vi "Create.vi"(8 "error in (no error)":errorcluster, 11 "Config XML":string) -> (0 "error out":errorcluster, 3 "reference out":refnum<class "ViPER.lvclass">)   [LabVIEW 2022 SP3, in "ViPER.lvlib" / "ViPER.lvclass"]
doc: "### BSD License (http://www.opensource.org/licenses/bsd-license.php) Begin ###\n\nCopyright (c) 2018 Kurt Friday www.medulla.net\n\nAll rights reserved.\n\nRedistribution and use in source and binary forms, with or without\nmodification, are permitted provided that the following conditions are met:\n\n * Redistributions of source code must retain the above copyright\n notice, this list of conditions and the following disclaimer.\n\n * Redistributions in binary form must reproduce the above copyright\n notice, this list of conditions and the following disclaimer in the\n documentation and/or other materials provided with the distribution.\n\n * Neither the name of the <organization> nor the\n names of its contributors may be used to endorse or promote products\n derived from this software without specific prior written permission.\n\nTHIS SOFTWARE IS PROVIDED BY THE COPYRIGHT HOLDERS AND CONTRIBUTORS \"AS IS\" AND\nANY EXPRESS OR IMPLIED WARRANTIES, INCLUDING, BUT NOT LIMITED TO, THE IMPLIED\nWARRANTIES OF MERCHANTABILITY AND FITNESS FOR A PARTICULAR PURPOSE ARE\nDISCLAIMED. IN NO EVENT SHALL <COPYRIGHT HOLDER> BE LIABLE FOR ANY\nDIRECT, INDIRECT, INCIDENTAL, SPECIAL, EXEMPLARY, OR CONSEQUENTIAL DAMAGES\n(INCLUDING, BUT NOT LIMITED TO, PROCUREMENT OF SUBSTITUTE GOODS OR SERVICES;\nLOSS OF USE, DATA, OR PROFITS; OR BUSINESS INTERRUPTION) HOWEVER CAUSED AND\nON ANY THEORY OF LIABILITY, WHETHER IN CONTRACT, STRICT LIABILITY, OR TORT\n(INCLUDING NEGLIGENCE OR OTHERWISE) ARISING IN ANY WAY OUT OF THE USE OF THIS\nSOFTWARE, EVEN IF ADVISED OF THE POSSIBILITY OF SUCH DAMAGE."
uses:
  ViPER.lvclass
  ObjectLayers.ctl
  <vilib>/Utility/LVLibp/NI_PackedLibraryUtility.lvlib
panel:
  # "### BSD License (http://www.opensource.org/licenses/bsd-license.php) Begin ###\n\nCopyright (c) 2018  Kurt Friday www.medulla.net\n\nAll rights reserved.\n\nRedistribution and use in source and binary forms, with or without\nmodification, are permitted provided that the following conditions are met:\n\n    * Redistributions of source code must retain the above copyright\n      notice, this list of conditions and the following disclaimer.\n\n    * Redistributions in binary form must reproduce the above copyright\n      notice, this list of conditions and the following disclaimer in the\n      documentation and/or other materials provided with the distribution.\n\n    * Neither the name of the <organization> nor the\n      names of its contributors may be used to endorse or promote products\n      derived from this software without specific prior written permission.\n\nTHIS SOFTWARE IS PROVIDED BY THE COPYRIGHT HOLDERS AND CONTRIBUTORS \"AS IS\" AND\nANY EXPRESS OR IMPLIED WARRANTIES, INCLUDING, BUT NOT LIMITED TO, THE IMPLIED\nWARRANTIES OF MERCHANTABILITY AND FITNESS FOR A PARTICULAR PURPOSE ARE\nDISCLAIMED. IN NO EVENT SHALL <COPYRIGHT HOLDER> BE LIABLE FOR ANY\nDIRECT, INDIRECT, INCIDENTAL, SPECIAL, EXEMPLARY, OR CONSEQUENTIAL DAMAGES\n(INCLUDING, BUT NOT LIMITED TO, PROCUREMENT OF SUBSTITUTE GOODS OR SERVICES;\nLOSS OF USE, DATA, OR PROFITS; OR BUSINESS INTERRUPTION) HOWEVER CAUSED AND\nON ANY THEORY OF LIABILITY, WHETHER IN CONTRACT, STRICT LIABILITY, OR TORT\n(INCLUDING NEGLIGENCE OR OTHERWISE) ARISING IN ANY WAY OUT OF THE USE OF THIS\nSOFTWARE, EVEN IF ADVISED OF THE POSSIBILITY OF SUCH DAMAGE."
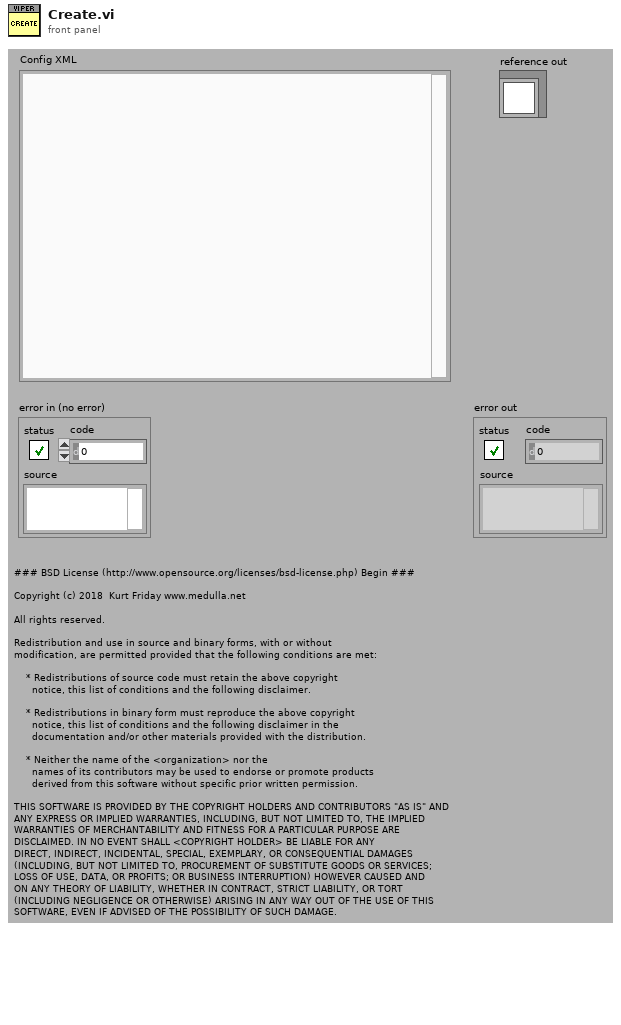
[diagram p1: front panel]
types:
  T1 = typedef "ViPER.lvlib/ViPER.lvclass/ObjectLayers.ctl" = cluster{"Ancestor":string, "Objects":refnum<class "ViPER.lvclass">[], "Object_Names":string[], "Owned":bool[]}
  T2 = typedef "ViPER.lvlib/ViPER.lvclass/ObjectDefinition.ctl" = cluster{"Name":string, "Ancestors":T3[]}
  T3 = typedef "ViPER.lvlib/ViPER.lvclass/Ancestor.ctl" = cluster{"Class":string, "Config":string, "Objects":string[]}
  T4 = typedef "ViPER.lvlib/ViPER.lvclass/Details.ctl" = cluster{"Name":string, "Class":string}
  T5 = typedef "ViPER.lvlib/ViPER.lvclass/ObjectAttributes.ctl" = cluster{"Object":T2, "Ancestors":T1[], "Config":T6, "Init_OK":bool, "Hierachy":string[], "PPL?":bool[], "SFP_Open":bool[], "Config_SFP_Open":bool[], "SoftFP_event":refnum<user-event>[], "ConfigFP_event":refnum<user-event>[], "SoftFP_Shutdown_Notifier":refnum<notifier>[], "ConfigFP_Shutdown_Notifier":refnum<notifier>[]}
  T6 = typedef "ViPER.lvlib/ViPER.lvclass/Config.ctl" = cluster{"default":string}
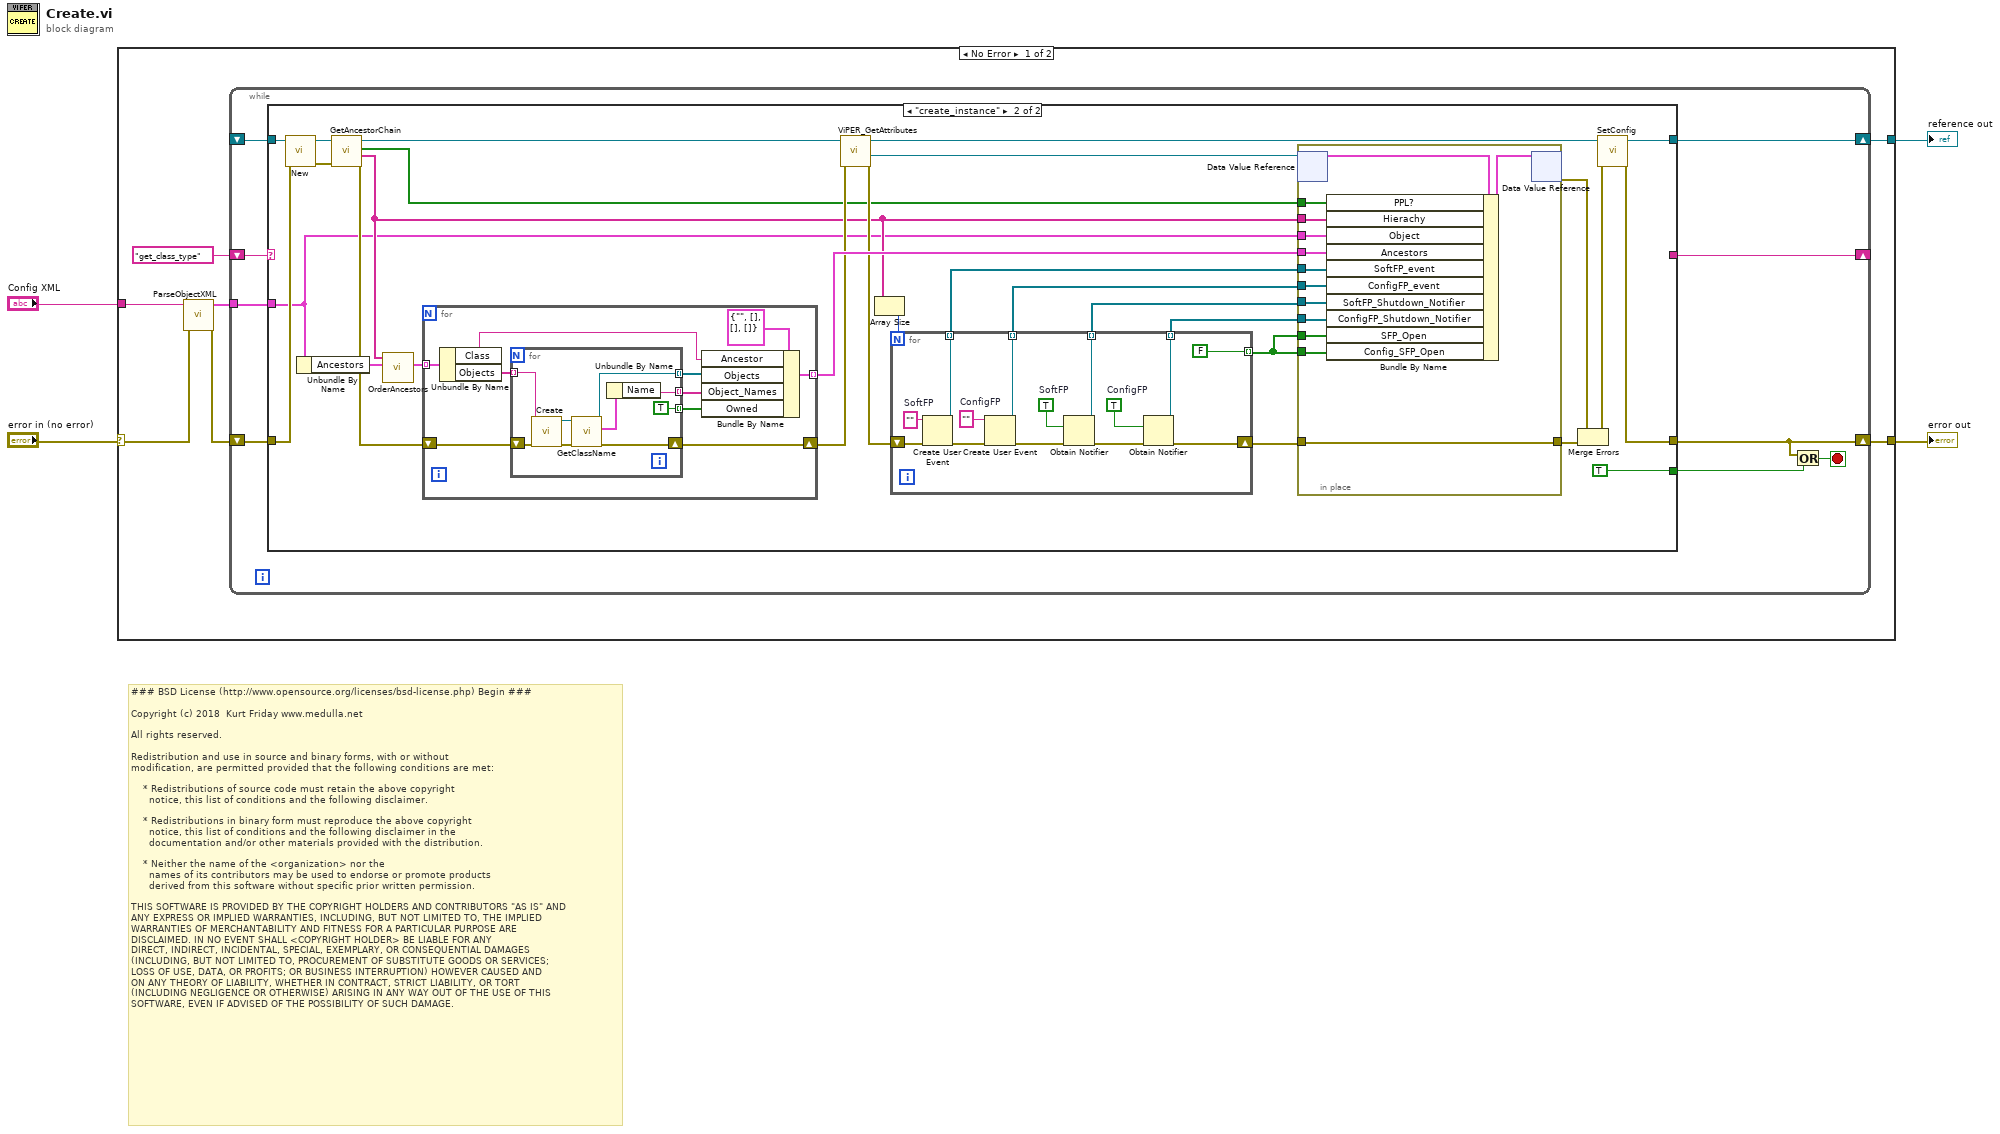
[diagram p0: block diagram]
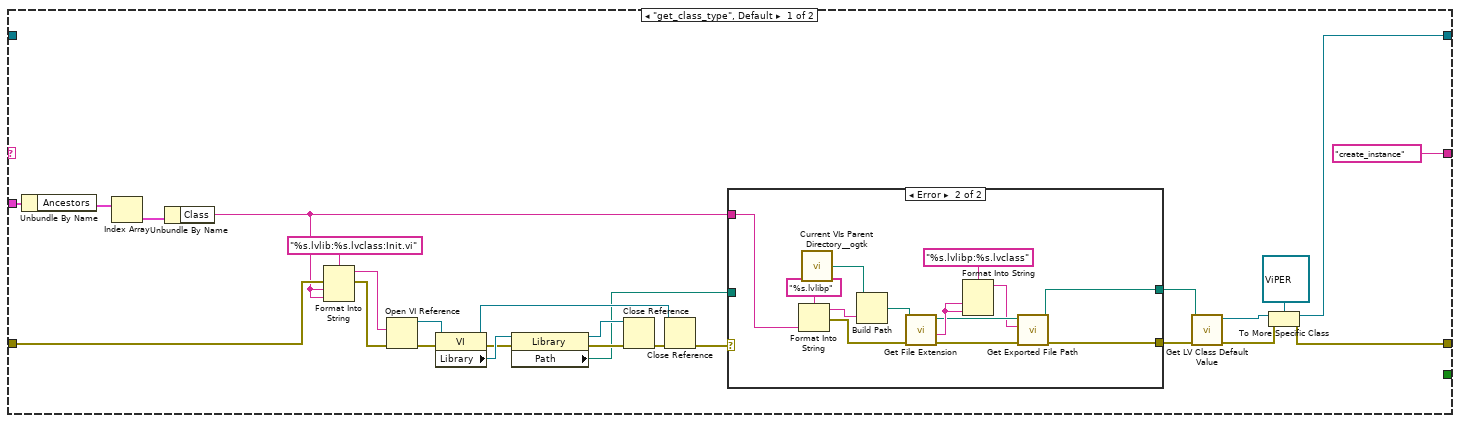
[diagram p2: hidden frame]
diagram:
  # "### BSD License (http://www.opensource.org/licenses/bsd-license.php) Begin ###\n\nCopyright (c) 2018  Kurt Friday www.medulla.net\n\nAll rights reserved.\n\nRedistribution and use in source and binary forms, with or without\nmodification, are permitted provided that the following conditions are met:\n\n    * Redistributions of source code must retain the above copyright\n      notice, this list of conditions and the following disclaimer.\n\n    * Redistributions in binary form must reproduce the above copyright\n      notice, this list of conditions and the following disclaimer in the\n      documentation and/or other materials provided with the distribution.\n\n    * Neither the name of the <organization> nor the\n      names of its contributors may be used to endorse or promote products\n      derived from this software without specific prior written permission.\n\nTHIS SOFTWARE IS PROVIDED BY THE COPYRIGHT HOLDERS AND CONTRIBUTORS \"AS IS\" AND\nANY EXPRESS OR IMPLIED WARRANTIES, INCLUDING, BUT NOT LIMITED TO, THE IMPLIED\nWARRANTIES OF MERCHANTABILITY AND FITNESS FOR A PARTICULAR PURPOSE ARE\nDISCLAIMED. IN NO EVENT SHALL <COPYRIGHT HOLDER> BE LIABLE FOR ANY\nDIRECT, INDIRECT, INCIDENTAL, SPECIAL, EXEMPLARY, OR CONSEQUENTIAL DAMAGES\n(INCLUDING, BUT NOT LIMITED TO, PROCUREMENT OF SUBSTITUTE GOODS OR SERVICES;\nLOSS OF USE, DATA, OR PROFITS; OR BUSINESS INTERRUPTION) HOWEVER CAUSED AND\nON ANY THEORY OF LIABILITY, WHETHER IN CONTRACT, STRICT LIABILITY, OR TORT\n(INCLUDING NEGLIGENCE OR OTHERWISE) ARISING IN ANY WAY OUT OF THE USE OF THIS\nSOFTWARE, EVEN IF ADVISED OF THE POSSIBILITY OF SUCH DAMAGE."
  n1 = case shown="No Error" "error in (no error)" {
    selector: "error in (no error)" -> [w8 w137]
    tunnel: "Config XML" -> [w9 _]
    tunnel: [w11 _] -> w1
    tunnel: [w10 w137] -> w2
    frame No Error {
      n2 = call "ParseObjectXML.vi"("error in (no error)"=w8, "Object XML"=w9) -> ("error out"=w7:errorcluster, "Object Cluster"=w5:T2)  [unwired: 8 in]
      n3 = while {
        shift-right: [w18] -> w10
        shift-left: w7 -> [w20]
        shift-right: [w17] -> w11
        shift-left: _ -> [w16]
        shift-right: [w15] -> _
        shift-left: "get_class_type" -> [w19]
        tunnel: w5 -> [w12]
        stop <- w13 stop-if-true
        n4 = case shown="\"create_instance\"" w19 {
          tunnel: w20 -> [w37 w84]
          tunnel: [w46 w68] -> w18
          tunnel: [w45 w70] -> w17
          tunnel: w16 -> [_ w86]
          tunnel: ["create_instance" _] -> w15
          tunnel: [_ TRUE] -> w14
          tunnel: w12 -> [w40 w64]
          frame "get_class_type", Default {
            n5 = Unbundle By Name(w40) -> ("Ancestors"=w39:T3[])
            n6 = Index Array(array=w39) -> (element=w38:T3)  [unwired: 1 in]
            n7 = Unbundle By Name(w38) -> ("Class"=w22:string)
            n8 = Format Into String(format string="%s.lvlib:%s.lvclass:Init.vi", error in=w37, w22, w22) -> (resulting string=w36:string, error out=w26:errorcluster)  [unwired: 1 in]
            n9 = Open VI Reference(vi path=w36, error in (no error)=w26) -> (vi reference=w33:refnum<vi>, error out=w28:errorcluster)  [unwired: 4 in]
            n10 = property class="VI"(reference=w33, error in=w28) -> (reference out=w35:refnum<vi>, error out=w29:errorcluster, "Library"=w30:refnum<vi>)
            n11 = property class="Library"(reference=w30, error in=w29) -> (reference out=w34:refnum<vi>, error out=w31:errorcluster, "Path"=w25:path)
            n12 = Close Reference(reference=w34, error in (no error)=w31) -> (error out=w32:errorcluster)
            n13 = Close Reference(reference=w35, error in (no error)=w32) -> (error out=w23:errorcluster)
            n14 = case shown="Error" w23 {
              selector: w23 -> [w47 _]
              tunnel: w25 -> [w48 _]
              tunnel: [w48 w50] -> w24
              tunnel: w22 -> [_ w51]
              tunnel: [w47 w49] -> w21
              frame No Error {
              }
              frame Error {
                n15 = Format Into String(format string="%s.lvlibp", w51) -> (resulting string=w60:string, error out=w54:errorcluster)  [unwired: 2 in]
                n16 = call <userlib>:"Current VIs Parent Directory__ogtk.vi"() -> ("Parent Directory (+ Relative)"=w59:path)  [unwired: 5 in]
                n17 = Build Path(base path=w59, name or relative path=w60) -> (appended path=w61:path)
                n18 = call <vilib>:"Get File Extension.vi"("error in (no error)"=w54, "file"=w61) -> ("error out"=w57:errorcluster, "filename without extension"=w58:string, "dup file"=w56:path)  [unwired: 5 in, 2 out]
                n19 = Format Into String(format string="%s.lvlibp:%s.lvclass", w58, w58) -> (resulting string=w55:string)  [unwired: 2 in, 1 out]
                n20 = call <vilib>:"Get Exported File Path.vi"("error in (no error)"=w57, "qualified name"=w55, "packed library path"=w56) -> ("error out"=w49:errorcluster, "path"=w50:path)  [unwired: 7 in]
              }
            }
            n21 = call <vilib>:"Get LV Class Default Value.vi"("error in (no error)"=w21, "class path"=w24) -> ("error out"=w41:errorcluster, "object"=w42:refnum<class>)  [unwired: 8 in]
            n22 = To More Specific Class(target class=refnum<class "ViPER.lvclass"> refnum ("reference out"), reference=w42, error in=w41) -> (specific class reference=w45:refnum<class "ViPER.lvclass">, error out=w46:errorcluster)
          }
          frame "create_instance" {
            n23 = call-dynamic "New.vi"("error in (no error)"=w84, "reference in"=w86) -> ("error out"=w74:errorcluster, "reference out"=w76:refnum<class "ViPER.lvclass">)  [unwired: 8 in]
            n24 = Unbundle By Name(w64) -> ("Ancestors"=w66:T3[])
            n25 = call-dynamic "GetAncestorChain.vi"("error in (no error)"=w74, "reference in"=w76) -> ("error out"=w73:errorcluster, "Chain Out"=w65:string[], "PPL? Out"=w72:bool[], "reference out"=w75:refnum<class "ViPER.lvclass">)  [unwired: 6 in]
            n26 = call "OrderAncestors.vi"("Ancestors in"=w66, "Ancestor Chain"=w65) -> ("Ancestors out"=w63:T3[])  [unwired: 9 in]
            n27 = for {
              shift-right: [w113] -> w78
              shift-left: w73 -> [w114]
              tunnel: w63 -> [w112] mode=indexing
              tunnel: [w107] -> w82 mode=indexing
              n28 = Unbundle By Name(w112) -> ("Class"=w109:string, "Objects"=w111:string[])
              n29 = for {
                shift-right: [w119] -> w113
                shift-left: w114 -> [w123]
                tunnel: w111 -> [w122] mode=indexing
                tunnel: [w117] -> w108 mode=indexing
                tunnel: [TRUE] -> w106 mode=indexing
                tunnel: [w115] -> w105 mode=indexing
                n30 = call "Create.vi"("error in (no error)"=w123, "Config XML"=w122) -> ("error out"=w120:errorcluster, "reference out"=w118:refnum<class "ViPER.lvclass">)  [unwired: 8 in]
                n31 = call "GetClassName.vi"("error in (no error)"=w120, "reference in"=w118) -> ("error out"=w119:errorcluster, "Details"=w116:T4, "reference out"=w117:refnum<class "ViPER.lvclass">)  [unwired: 7 in]
                n32 = Unbundle By Name(w116) -> ("Name"=w115:string)
              }
              n33 = Bundle By Name(cluster=T1 {"Ancestor"="", "Objects"=[], "Object_Names"=[], "Owned"=[]} ("Layer"), "Ancestor"=w109, "Objects"=w108, "Object_Names"=w105, "Owned"=w106) -> (w107:T1)
            }
            n34 = call "ViPER_GetAttributes.vi"("error in (no error)"=w78, "reference in"=w75) -> ("error out"=w77:errorcluster, "DataRef"=w83:refnum<data-value>, "reference out"=w71:refnum<class "ViPER.lvclass">)  [unwired: 6 in, 1 out]
            n35 = Array Size(array=w65) -> (size(s)=w67:i32)
            n36 = for {
              N: w67 -> [_]
              tunnel: [w101] -> w88 mode=indexing
              tunnel: [w100] -> w87 mode=indexing
              tunnel: [w98] -> w81 mode=indexing
              tunnel: [w95] -> w80 mode=indexing
              shift-right: [w91] -> w79
              shift-left: w77 -> [w94]
              tunnel: [FALSE] -> w62 mode=indexing
              w96 = TRUE  # ConfigFP
              w99 = TRUE  # SoftFP
              w103 = ""  # ConfigFP
              w104 = ""  # SoftFP
              n37 = Create User Event(user event datatype=w104, error in=w94) -> (user event=w101:refnum<user-event>, error out=w102:errorcluster)
              n38 = Create User Event(user event datatype=w103, error in=w102) -> (user event=w100:refnum<user-event>, error out=w92:errorcluster)
              n39 = Obtain Notifier(notification data type=w99, error in (no error)=w92) -> (notifier out=w98:refnum<notifier>, error out=w97:errorcluster)  [unwired: 2 in, 1 out]
              n40 = Obtain Notifier(notification data type=w96, error in (no error)=w97) -> (notifier out=w95:refnum<notifier>, error out=w91:errorcluster)  [unwired: 2 in, 1 out]
            }
            n41 = in-place {
              in-place-border: w79 -> [w134]
              in-place-border: [w134] -> w89
              in-place-border: w64 -> [w129]
              in-place-border: w88 -> [w133]
              in-place-border: w87 -> [w132]
              in-place-border: w81 -> [w131]
              in-place-border: w80 -> [w130]
              in-place-border: w82 -> [w128]
              in-place-border: w65 -> [w127]
              in-place-border: w72 -> [w126]
              in-place-border: w62 -> [w125]
              in-place-border: w62 -> [w124]
              n42 = in-place-dvr #1(w83) -> (w135:T5)  [unwired: 1 out]
              n43 = Bundle By Name(cluster=w135, "PPL?"=w126, "Hierachy"=w127, "Object"=w129, "Ancestors"=w128, "SoftFP_event"=w133, "ConfigFP_event"=w132, "SoftFP_Shutdown_Notifier"=w131, "ConfigFP_Shutdown_Notifier"=w130, "SFP_Open"=w125, "Config_SFP_Open"=w124) -> (w136:T5)
              n44 = in-place-dvr #1(w136) -> (w90:errorcluster)  [unwired: 1 out]
            }
            n45 = Merge Errors(w90, w89) -> (w69:errorcluster)
            n46 = call-dynamic "SetConfig.vi"("error in (no error)"=w69, "reference in"=w71) -> ("error out"=w68:errorcluster, "reference out"=w70:refnum<class "ViPER.lvclass">)  [unwired: 8 in]
          }
        }
        n47 = Or(x=w18, y=w14) -> (x .or. y?=w13:bool)
      }
    }
    frame Error {
    }
  }
  "error out" <- w2
  "reference out" <- w1
